vi "To String.vi"(11 "JSON Numeric in":refnum<class "JSON Numeric.lvclass">) -> (2 "String":string)   [LabVIEW 2017, in "LVJSON.lvlib" / "JSON Numeric.lvclass"]
uses:
  JSON Numeric.lvclass
  JSON Numeric.lvclass/JSON Numeric.ctl
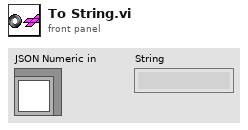
[diagram p1: front panel]
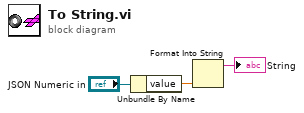
[diagram p0: block diagram]
diagram:
  n1 = Unbundle By Name("JSON Numeric in") -> ("value"=w2:dbl)
  n2 = Format Into String(w2) -> (resulting string=→"String":string)  [unwired: 3 in, 1 out]
